vi "MaximizeFrontPanelTest2.vi"() -> ()   [LabVIEW 2018]
uses:
  System.Windows.Forms
  System.Drawing
panel:
  out "Array":cluster{"Width":i32, "Height":i32}[](array[cluster])
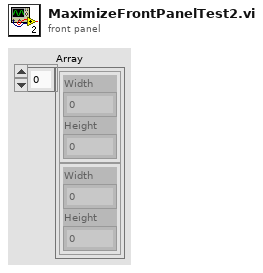
[diagram p1: front panel]
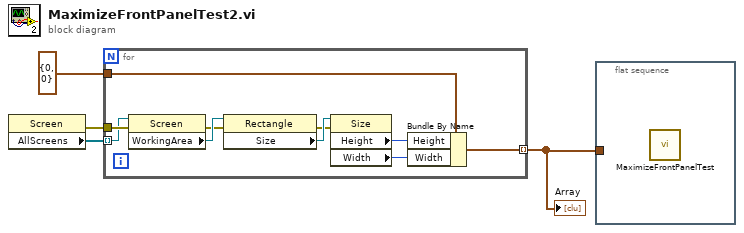
[diagram p0: block diagram]
diagram:
  n1 = property class="Screen"() -> (error out=w3:errorcluster, "AllScreens"=w4:refnum<k24>[])  [unwired: 2 in, 1 out]
  n2 = for {
    tunnel: w4 -> [w5] mode=indexing
    tunnel: w3 -> [w13]
    tunnel: [w8] -> w2 mode=indexing
    tunnel: cluster{"Width":i32, "Height":i32} {"Width"=0, "Height"=0} -> [w6]
    n3 = property class="Screen"(reference=w5, error in=w13) -> (error out=w12:errorcluster, "WorkingArea"=w14:refnum<k24>)  [unwired: 1 out]
    n4 = property class="Rectangle"(reference=w14, error in=w12) -> (error out=w10:errorcluster, "Size"=w11:refnum<k24>)  [unwired: 1 out]
    n5 = property class="Size"(reference=w11, error in=w10) -> ("Height"=w9:i32, "Width"=w7:i32)  [unwired: 2 out]
    n6 = Bundle By Name(cluster=w6, "Height"=w9, "Width"=w7) -> (w8:cluster{"Width":i32, "Height":i32})
  }
  "Array" <- w2
  n7 = flat-sequence {
    tunnel: w2 -> [_]
    frame #0 {
      n8 = call "MaximizeFrontPanelTest.vi"() -> ()  [unwired: 12 in]
    }
  }
